vi "Reset Device to Default State.vi"(8 "error in (no error)":errorcluster, 11 "VISA resource name":refnum<visa-resource-name>) -> (0 "error out":errorcluster, 3 "VISA resource name out":refnum<visa-resource-name>)   [LabVIEW 2013, in "SRS SR400.lvlib"]
doc: "<B>CL</B>\n\nThe CL command resets the unit to its default state. The default front panel settings are listed in the Instrument Setups section. Parameters in the SETUP and COM menus are not changed. In addition, the SRQ mask is cleared, and the RS-232 terminating sequence is reset to the proper defaults.\n\nThe command and output buffers are cleared by the CL command. Therefore, it is bad practice to use the CL command before all previous commands have been processed and all responses have been received. There should never be any other commands on the same line as a CL command."
uses:
  <instrlib>/SRS SR400/SRS SR400.lvlib
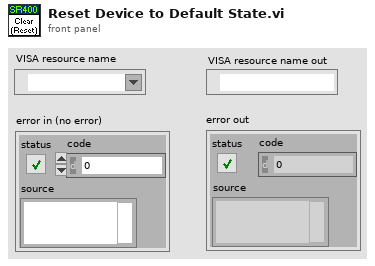
[diagram p1: front panel]
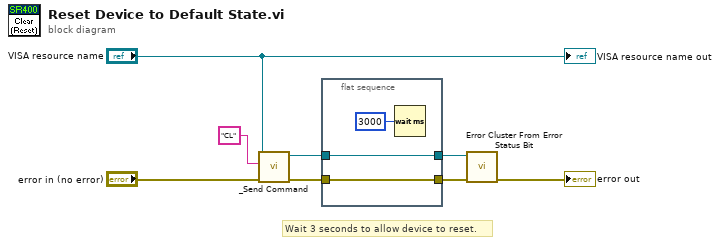
[diagram p0: block diagram]
diagram:
  # "Wait 3 seconds to allow device to reset."
  n1 = call <instrlib>:"_Send Command.vi"("error in (no error)"="error in (no error)", "Command"="CL" ("command"), "VISA resource name"="VISA resource name") -> ("error out"=w2:errorcluster, "VISA resource name out"=w4:refnum<visa-resource-name>)  [unwired: 1 in, 6 out]
  n2 = flat-sequence {
    tunnel: [w11] -> w3
    tunnel: w4 -> [w11]
    tunnel: [w10] -> w1
    tunnel: w2 -> [w10]
    frame #0 {
      n3 = Wait (ms)(milliseconds to wait=u32 3000) -> ()  [unwired: 1 out]
    }
  }
  n4 = call <instrlib>:"Error Cluster From Error Status Bit.vi"("error in (no error)"=w1, "VISA resource name"=w3) -> ("error out"=→"error out":errorcluster)  [unwired: 8 in, 1 out]
  "VISA resource name out" <- "VISA resource name"
